vi "Generate version file.vi"(8 "error in (no error)":errorcluster, 11 "Project Path":path=path "C:/LabVIEW Code/TALOS/talos/TALOS.lvproj") -> (0 "error out":errorcluster)   [LabVIEW 2026]
uses:
  <vilib>/Utility/error.llb/Trim Whitespace (string).vi
  <vilib>/Utility/error.llb/Trim Whitespace One-Sided.vi
panel:
  out "standard output 2":string
  out "standard error":string
  out "standard output":string
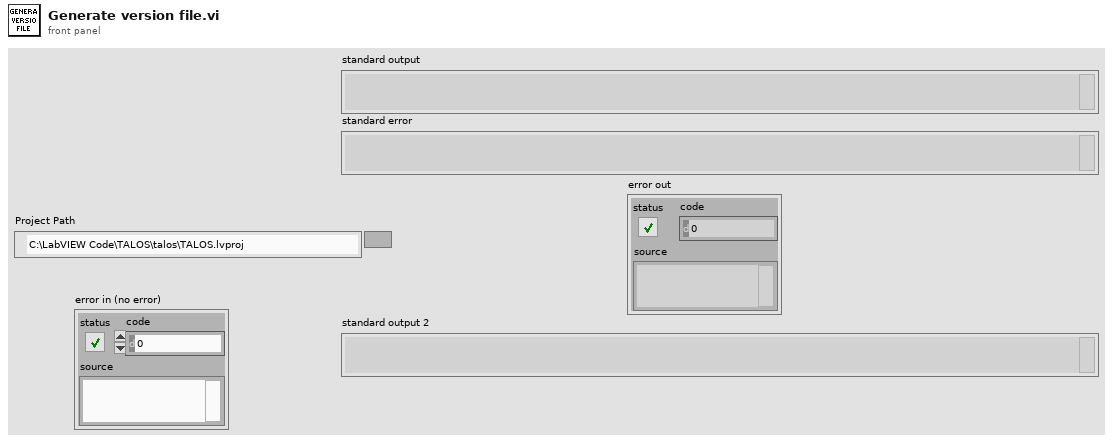
[diagram p1: front panel]
types:
  T1 = enum16{"open", "replace", "create", "open or create", "replace or create", "replace or create with confirmation"}
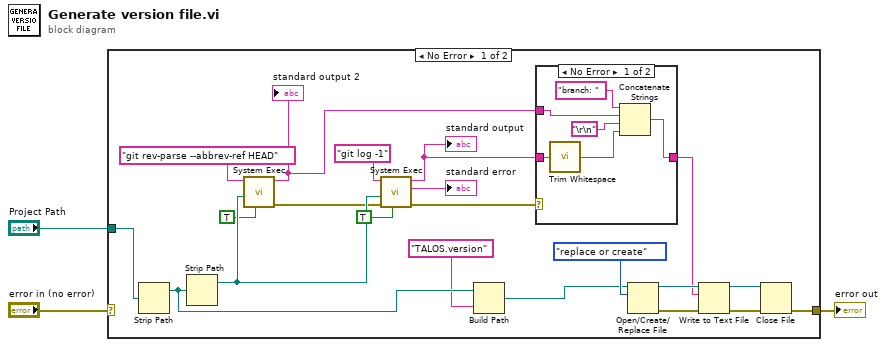
[diagram p0: block diagram]
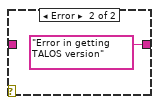
[diagram p2: hidden frame]
diagram:
  n1 = case shown="No Error" "error in (no error)" {
    selector: "error in (no error)" -> [_ w32]
    tunnel: "Project Path" -> [w24 _]
    tunnel: [w13 w32] -> w2
    frame No Error {
      n2 = Strip Path(path=w24) -> (stripped path=w11:path)  [unwired: 1 out]
      n3 = Strip Path(path=w11) -> (stripped path=w9:path)  [unwired: 1 out]
      n4 = call <vilib>:"System Exec.vi"("run minimized? (F)"=TRUE, "working directory"=w9, "command line"="git rev-parse --abbrev-ref HEAD") -> ("error out"=w8:errorcluster, "standard output"=w6:string)  [unwired: 5 in, 2 out]
      "standard output 2" <- w6
      n5 = call <vilib>:"System Exec.vi"("run minimized? (F)"=TRUE, "error in (no error)"=w8, "working directory"=w9, "command line"="git log -1") -> ("error out"=w21:errorcluster, "standard error"=→"standard error":string, "standard output"=w15:string)  [unwired: 4 in, 1 out]
      "standard output" <- w15
      n6 = Build Path(base path=w11, name or relative path="TALOS.version") -> (appended path=w12:path)
      n7 = case shown="No Error" w21 {
        tunnel: w15 -> [w30 _]
        tunnel: [w25 "Error in getting TALOS version" ("trimmed string")] -> w14
        tunnel: w6 -> [w28 _]
        frame No Error {
          n8 = call-poly <vilib>:"Trim Whitespace.vi"("string"=w30) -> ("trimmed string"=w26:string)  [unwired: 1 in]
          n9 = Concatenate Strings("branch: " ("string"), w28, "\r\n", w26) -> (w25:string)
        }
        frame Error {
        }
      }
      n10 = Open/Create/Replace File(file path (use dialog)=w12, operation (0:open)=T1."replace or create") -> (refnum out=w16:refnum<file>, error out=w20:errorcluster)  [unwired: 4 in, 1 out]
      n11 = Write to Text File(file (use dialog)=w16, text=w14, error in=w20) -> (refnum out=w18:refnum<file>, error out=w19:errorcluster)  [unwired: 1 in, 1 out]
      n12 = Close File(refnum=w18, error in=w19) -> (error out=w13:errorcluster)  [unwired: 1 out]
    }
    frame Error {
    }
  }
  "error out" <- w2
